vi "Create.vi"(8 "error in (no error)":errorcluster, 9 "Distance":u64, 10 "Time":u64) -> (0 "error out":errorcluster, 3 "Race Out":refnum<class "Race.lvclass">)   [LabVIEW 2021, in "Race.lvclass"]
uses:
  Race.lvclass
  Race.lvclass/Race.ctl
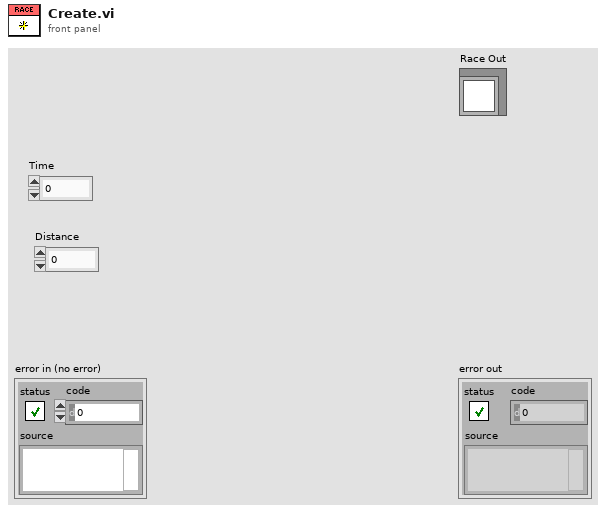
[diagram p1: front panel]
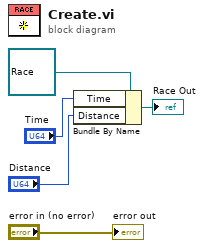
[diagram p0: block diagram]
diagram:
  n1 = Bundle By Name(cluster=refnum<class "Race.lvclass"> refnum ("Race"), "Time"="Time", "Distance"="Distance") -> (→"Race Out":refnum<class "Race.lvclass">)
  "error out" <- "error in (no error)"
